vi "Set System Explorer Busy.vi"(8 "error in":errorcluster) -> (0 "error out":errorcluster)   [LabVIEW 2020, in "Ballard MIL-STD-1553 System Explorer.lvlib" / "Implementation.lvlib"]
uses:
  Implementation.lvlib
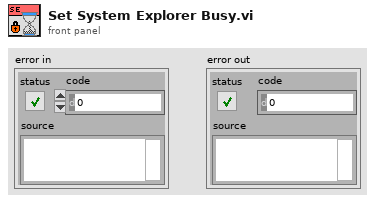
[diagram p1: front panel]
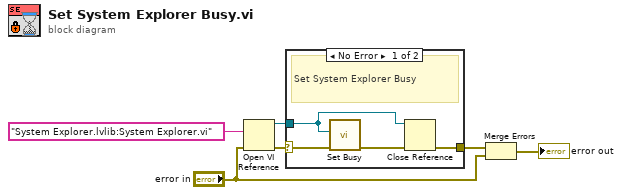
[diagram p0: block diagram]
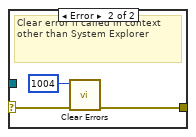
[diagram p2: hidden frame]
diagram:
  n1 = Open VI Reference(vi path="System Explorer.lvlib:System Explorer.vi", error in (no error)="error in") -> (vi reference=w4:refnum<vi>, error out=w5:errorcluster)  [unwired: 4 in]
  n2 = case shown="No Error" w5 {
    selector: w5 -> [w10 w13]
    tunnel: w4 -> [w8 _]
    tunnel: [w7 w12] -> w2
    frame No Error {
      # "Set System Explorer Busy"
      n3 = call <vilib>:"Set Busy.vi"("error in (no error)"=w10, "VI reference (current VI)"=w8) -> ("error out"=w9:errorcluster)  [unwired: 8 in, 1 out]
      n4 = Close Reference(reference=w8, error in (no error)=w9) -> (error out=w7:errorcluster)
    }
    frame Error {
      # "Clear error if called in context other than System Explorer"
      n5 = call <vilib>:"Clear Errors.vi"("error in (no error)"=w13, "specific error code to clear (0: all)"=1004) -> ("error out"=w12:errorcluster)  [unwired: 4 in, 1 out]
    }
  }
  n6 = Merge Errors(w2, "error in") -> (→"error out":errorcluster)
